vi "WriterDaemon.vi"(8 "error in (no error)":errorcluster, 10 "Variant Queue":refnum<queue>, 11 "Writer Endpoint":refnum<k21>) -> ()   [LabVIEW 2011, in "NetworkStreamWriter.lvclass"]
doc: "Daemon (running in the background) which consistently checks the internal queue to see if a new value is available. If a new value is available, it is written across the network stream."
uses:
  NetworkStreamWriter.lvclass
  2-Think/2 Globals/2 Global.vi
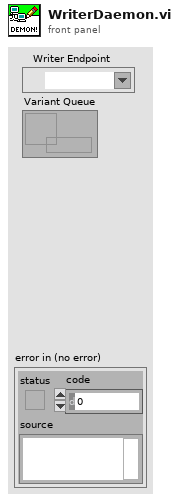
[diagram p1: front panel]
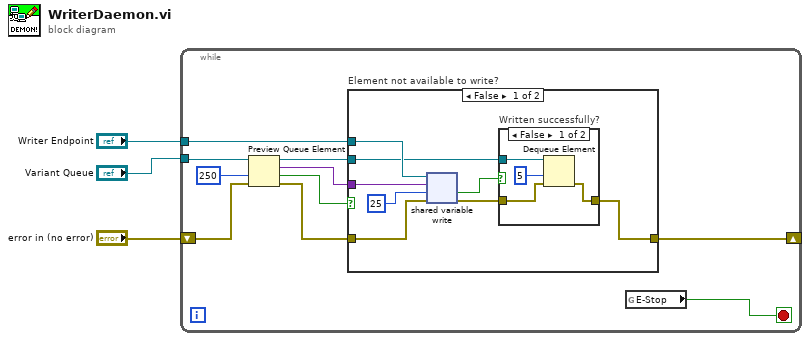
[diagram p0: block diagram]
diagram:
  n1 = while {
    tunnel: "Writer Endpoint" -> [w7]
    tunnel: "Variant Queue" -> [w13]
    shift-right: [w5] -> _
    shift-left: "error in (no error)" -> [w12]
    stop <- w4 stop-if-true
    n2 = Preview Queue Element(queue=w13, timeout in ms (-1)=250, error in (no error)=w12) -> (queue out=w6:refnum<queue>, element=w9:variant, timed out?=w10:bool, error out=w8:errorcluster)
    n3 = case "Element not available to write?" shown="False" w10 {
      tunnel: w9 -> [w20 _]
      tunnel: w8 -> [w19 w27]
      tunnel: w7 -> [w21 _]
      tunnel: w6 -> [w18 _]
      tunnel: [w16 w27] -> w5
      frame False {
        n4 = shared-variable-write(w21, w19, w20, 25 ("timeout ms (-1)")) -> (w17:errorcluster, w14:bool)  [unwired: 1 out]
        n5 = case "Written successfully?" shown="False" w14 {
          tunnel: w18 -> [w25 _]
          tunnel: w17 -> [w24 w26]
          tunnel: [w22 w26] -> w16
          frame False {
            n6 = Dequeue Element(queue=w25, timeout in ms (-1)=5, error in (no error)=w24) -> (error out=w22:errorcluster)  [unwired: 3 out]
          }
          frame True {
          }
        }
      }
      frame True {
      }
    }
    n7 = global read "2 Global.vi" "E-Stop"() -> (w4:bool)
  }
